vi "Config FFT.vi"(0 "VISA resource name":refnum<visa-resource-name>, 5 "FFT Points (0: 1000)":u16(ring) items=["1000", "2000", "10000"], 7 "FFT Window (0: Rect)":u16(ring) items=["Rect", "Hanning"], 11 "error in (no error)":errorcluster) -> (4 "VISA resource name out":refnum<visa-resource-name>, 15 "error out":errorcluster)   [LabVIEW 2013, in "Yokogawa.lvlib" / "Yokogawa PZ4000.lvlib"]
doc: "This VI sends the Math command to the PZ4000 series.\nConfigure Control Functions are Selects the FFT Points and FFT WIndow."
uses:
  Yokogawa PZ4000.lvlib
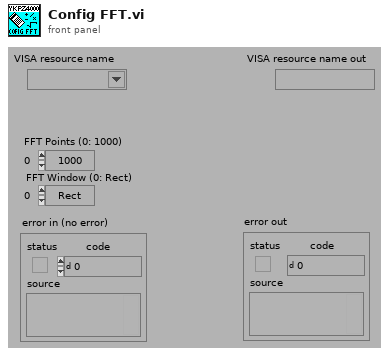
[diagram p1: front panel]
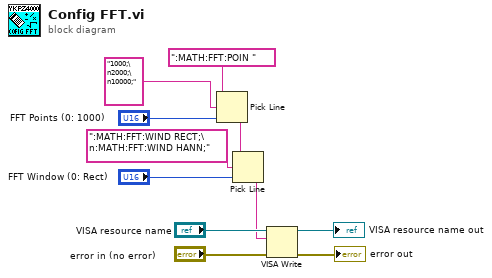
[diagram p0: block diagram]
diagram:
  n1 = Pick Line(string ("")=":MATH:FFT:POIN ", multi-line string="1000;\n2000;\n10000;", line index="FFT Points (0: 1000)") -> (output string=w1:string)
  n2 = Pick Line(string ("")=w1, multi-line string=":MATH:FFT:WIND RECT;\n:MATH:FFT:WIND HANN;", line index="FFT Window (0: Rect)") -> (output string=w2:string)
  n3 = VISA Write(VISA resource name="VISA resource name", write buffer=w2, error in (no error)="error in (no error)") -> (VISA resource name out=→"VISA resource name out":refnum<visa-resource-name>, error out=→"error out":errorcluster)  [unwired: 1 out]
